vi "DrumSeq_Pulsed_Multiple_Example.vi"() -> ()   [LabVIEW 2019]
uses:
  <vilib>/Rock Robotics/WPI/ThirdParty/JAS_Junk/TrajLib/Enum/AutoHelperSequence_Step_Enum.ctl
  <vilib>/Rock Robotics/WPI/ThirdParty/JAS_Junk/TrajLib/VI/Util_GetTime_U32.vi
  <vilib>/Rock Robotics/WPI/ThirdParty/JAS_Junk/TrajLib/VI/BoolCmd_Recv_Internal.vi
  <vilib>/Rock Robotics/WPI/ThirdParty/JAS_Junk/TrajLib/Timer_New.vi
  <vilib>/Rock Robotics/WPI/ThirdParty/JAS_Junk/TrajLib/VI/BoolCmd_Send_Internal.vi
  <vilib>/Rock Robotics/WPI/ThirdParty/JAS_Junk/TrajLib/VI/BoolCmd_ObtainQueue.vi
  <vilib>/Rock Robotics/WPI/ThirdParty/JAS_Junk/TrajLib/VI/Util_GetTime_U64.vi
  <vilib>/Utility/semaphor.llb/Obtain Semaphore Reference.vi
  <vilib>/Rock Robotics/WPI/ThirdParty/JAS_Junk/TrajLib/Timer_Reset.vi
  <vilib>/Rock Robotics/WPI/ThirdParty/JAS_Junk/TrajLib/VI/Timer_Restart.vi
  <vilib>/Rock Robotics/WPI/ThirdParty/JAS_Junk/TrajLib/Timer_HasPeriodPassedOnce.vi
  <vilib>/Rock Robotics/WPI/ThirdParty/JAS_Junk/TrajLib/Trajectory_Library.lvlib
panel:
  in  "Teleop Action\nCancel":bool
  out "Auto Step Number":T1
  out "Auto\nActive":bool
  in  "Start\nAutonomous":bool
  in  "Teleop Action\nCapture":bool
  in  "Teleop Action\nRelease":bool
  out "Hand Control \nOutput":bool
  out "Waveform Chart":cluster{i16, i16}(graph)
  out "Arm Control\nOutput":bool
  # "PULSED DRUM SEQUENCER - MULTIPLE"
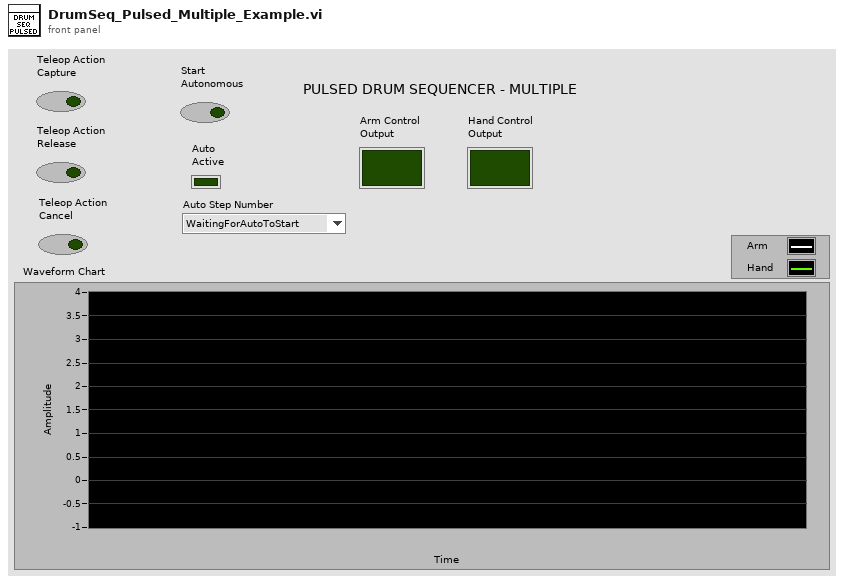
[diagram p1: front panel]
types:
  T1 = typedef "Trajectory_Library.lvlib/AutoHelperSequence_Step_Enum.ctl" = enum16{"WaitingForAutoToStart", "Step 1", "Step 2", "Step 3", "Step 4", "Step 5", "Step 6", "Step 7", "Step 8", "Step 9", "Step 10", "Step 11", "Step 12", "Step 13", "Step 14", "Step 15", "Step 16", "Step 17", "Step 18", "Step 19", "Step 20", "Step 21", "Step 22", "Step 23", "Step 24", "Step 25", "Step 26", "Step 27", "Step 28", "Step 29", "Step 30", "Step 31", "Step 32", "AutoDone"}
  T2 = typedef "Trajectory_Library.lvlib/DrumSequence_Step_Enum.ctl" = enum16{"Do Nothing", "Step 1", "Step 2", "Step 3", "Step 4", "Step 5", "Step 6", "Step 7", "Step 8", "Step 9", "Step 10", "Step 11", "Step 12", "Step 13", "Step 14", "Step 15", "Step 16", "Step 17", "Step 18", "Step 19", "Step 20", "Step 21", "Step 22", "Step 23", "Step 24", "Step 25", "Step 26", "Step 27", "Step 28", "Step 29", "Step 30", "Step 31", "Step 32", "Cancel", "Initialize", "Error"}
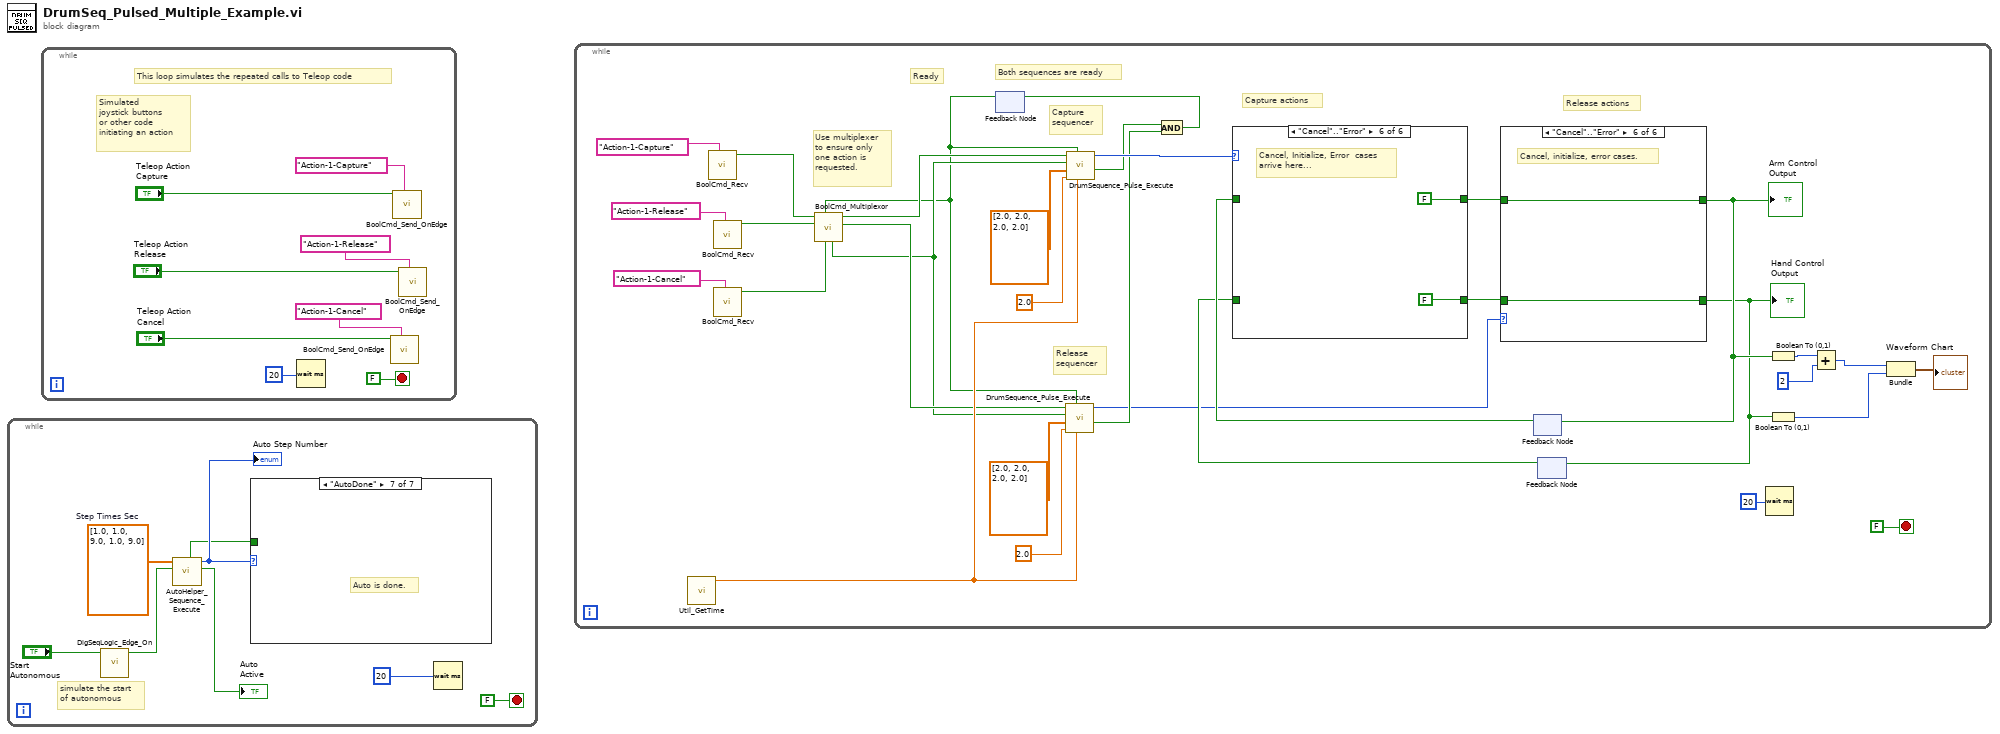
[diagram p0: block diagram]
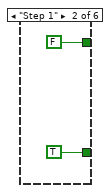
[diagram p3: hidden frame]
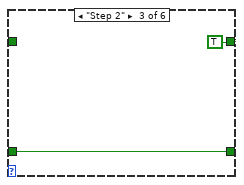
[diagram p4: hidden frame]
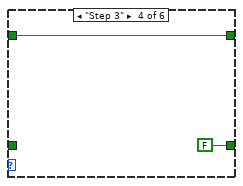
[diagram p5: hidden frame]
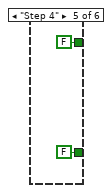
[diagram p6: hidden frame]
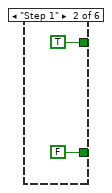
[diagram p8: hidden frame]
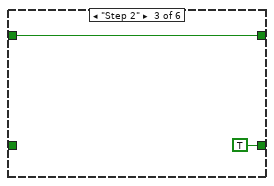
[diagram p9: hidden frame]
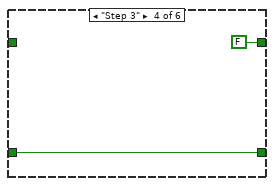
[diagram p10: hidden frame]
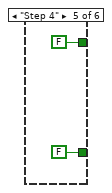
[diagram p11: hidden frame]
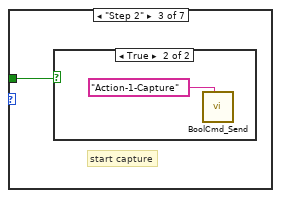
[diagram p14: hidden frame]
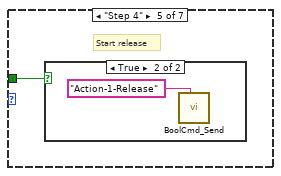
[diagram p17: hidden frame]
diagram:
  n1 = while {
    stop <- FALSE stop-if-true
    w5 = dbl[] [1.0, 1.0, 9.0, 1.0, 9.0]  # Step Times Sec
    # "simulate the start\nof autonomous"
    n2 = call <vilib>:"DigSeqLogic_Edge_On.vi"("Input"="Start\nAutonomous") -> ("On Edge"=w4:bool)  [unwired: 10 in]
    n3 = call <vilib>:"AutoHelper_Sequence_Execute.vi"("Initiate"=w4, "Step Times Sec"=w5) -> ("Seq  Active"=→"Auto\nActive":bool, "Step Number State"=w3:T1, "New Step"=w2:bool)  [unwired: 5 in, 2 out]
    "Auto Step Number" <- w3
    n4 = case shown="\"AutoDone\"" w3 {
      tunnel: w2 -> [_ _ w9 _ w11 _ _]
      frame "WaitingForAutoToStart", Default {
        # "do nothing"
      }
      frame "Step 1" {
        # "do nothing"
      }
      frame "Step 2" {
        # "start capture"
        n5 = case shown="True" w9 {
          frame False {
          }
          frame True {
            n6 = call <vilib>:"BoolCmd_Send.vi"("Command Name"="Action-1-Capture") -> ()  [unwired: 10 in, 1 out]
          }
        }
      }
      frame "Step 3" {
        # "Do nothing"
      }
      frame "Step 4" {
        # "Start release"
        n7 = case shown="True" w11 {
          frame False {
          }
          frame True {
            n8 = call <vilib>:"BoolCmd_Send.vi"("Command Name"="Action-1-Release") -> ()  [unwired: 10 in, 1 out]
          }
        }
      }
      frame "Step 5" {
        # "Do nothing"
      }
      frame "AutoDone" {
        # "Auto is done."
      }
    }
    n9 = Wait (ms)(milliseconds to wait=u32 20 ("milliseconds to wait 2")) -> ()  [unwired: 1 out]
  }
  n10 = while {
    stop <- FALSE stop-if-true
    # "Simulated\njoystick buttons\nor other code \ninitiating an action"
    # "This loop simulates the repeated calls to Teleop code"
    n11 = Wait (ms)(milliseconds to wait=u32 20) -> ()  [unwired: 1 out]
    n12 = call <vilib>:"BoolCmd_Send_OnEdge.vi"("Command Name"="Action-1-Cancel", "Value"="Teleop Action\nCancel") -> ()  [unwired: 9 in, 1 out]
    n13 = call <vilib>:"BoolCmd_Send_OnEdge.vi"("Command Name"="Action-1-Capture", "Value"="Teleop Action\nCapture") -> ()  [unwired: 9 in, 1 out]
    n14 = call <vilib>:"BoolCmd_Send_OnEdge.vi"("Command Name"="Action-1-Release", "Value"="Teleop Action\nRelease") -> ()  [unwired: 9 in, 1 out]
  }
  n15 = while {
    stop <- FALSE stop-if-true
    # "Use multiplexer\nto ensure only\none action is\nrequested."
    # "Ready"
    # "Release actions"
    # "Capture actions"
    # "Both sequences are ready"
    # "Release\nsequencer"
    # "Capture\nsequencer"
    n16 = call <vilib>:"Util_GetTime.vi"() -> ("FPGA_Time_Seconds"=w36:dbl)  [unwired: 9 in, 2 out]
    n17 = call <vilib>:"BoolCmd_Recv.vi"("Command Name"="Action-1-Capture") -> ("New Request"=w31:bool)  [unwired: 9 in, 1 out]
    n18 = call <vilib>:"BoolCmd_Recv.vi"("Command Name"="Action-1-Release") -> ("New Request"=w30:bool)  [unwired: 9 in, 1 out]
    n19 = call <vilib>:"BoolCmd_Recv.vi"("Command Name"="Action-1-Cancel") -> ("New Request"=w29:bool)  [unwired: 9 in, 1 out]
    n20 = feedback #1() -> (w32:bool)  [unwired: 1 in]
    n21 = call <vilib>:"BoolCmd_Multiplexor.vi"("Command Cancel"=w29, "Ready"=w32, "Command 2"=w30, "Command 1"=w31) -> ("Do Command 2"=w34:bool, "Do Command 1"=w35:bool, "Do Cancel"=w33:bool)  [unwired: 3 in, 2 out]
    n22 = call <vilib>:"DrumSequence_Pulse_Execute.vi"("Pass_Through_Time"=w36, "External Ready"=w32, "Cancel Time Sec"=2.0, "Step Times Sec"=dbl[] [2.0, 2.0, 2.0, 2.0], "Cancel"=w33, "Initiate"=w34) -> ("Ready"=w39:bool, "Step Number State"=w37:T2)  [unwired: 2 in, 2 out]
    n23 = call <vilib>:"DrumSequence_Pulse_Execute.vi"("Pass_Through_Time"=w36, "External Ready"=w32, "Cancel Time Sec"=2.0, "Step Times Sec"=dbl[] [2.0, 2.0, 2.0, 2.0], "Cancel"=w33, "Initiate"=w35) -> ("Ready"=w40:bool, "Step Number State"=w47:T2)  [unwired: 2 in, 2 out]
    n24 = And(x=w40, y=w39) -> (x .and. y?=w38:bool)
    n25 = feedback-in #1(w38) -> ()
    n26 = feedback #2() -> (w46:bool)  [unwired: 1 in]
    n27 = feedback #3() -> (w45:bool)  [unwired: 1 in]
    n28 = case shown="\"Cancel\"..\"Error\"" w47 {
      tunnel: [w67 TRUE w70 FALSE FALSE FALSE] -> w44
      tunnel: [w66 FALSE TRUE w72 FALSE FALSE] -> w43
      tunnel: w46 -> [w67 _ w70 _ _ _]
      tunnel: w45 -> [w66 _ _ w72 _ _]
      frame "Do Nothing", Default {
      }
      frame "Step 1" {
      }
      frame "Step 2" {
      }
      frame "Step 3" {
      }
      frame "Step 4" {
      }
      frame "Cancel".."Error" {
        # "Cancel, Initialize, Error  cases\narrive here..."
      }
    }
    n29 = case shown="\"Cancel\"..\"Error\"" w37 {
      tunnel: [w55 FALSE TRUE w61 FALSE w65] -> w22
      tunnel: [w54 TRUE w58 FALSE FALSE w64] -> w21
      tunnel: w44 -> [w55 _ _ w61 _ w65]
      tunnel: w43 -> [w54 _ w58 _ _ w64]
      frame "Do Nothing", Default {
      }
      frame "Step 1" {
      }
      frame "Step 2" {
      }
      frame "Step 3" {
      }
      frame "Step 4" {
      }
      frame "Cancel".."Error" {
        # "Cancel, initialize, error cases."
      }
    }
    "Arm Control\nOutput" <- w22
    "Hand Control \nOutput" <- w21
    n30 = feedback-in #2(w22) -> ()
    n31 = feedback-in #3(w21) -> ()
    n32 = Wait (ms)(milliseconds to wait=u32 20) -> ()  [unwired: 1 out]
    n33 = Boolean To (0,1)(Boolean=w22) -> (0, 1=w26:i16)
    n34 = Boolean To (0,1)(Boolean=w21) -> (0, 1=w24:i16)
    n35 = Add(x=w26, y=i16 2) -> (x+y=w25:i16)
    n36 = Bundle(w25, w24) -> (→"Waveform Chart":cluster{i16, i16})  [unwired: 1 in]
  }
